vi "CONV 2D String Array to String.vi"(0 "2-D String":string[][](array[string]), 1 "Delimiters (,;)":string=",;") -> (6 "String":string)   [LabVIEW 2017]
doc: "This routine converts a 2-D String Array into a String list. There must be exactly 2 characters in the delimiters field. The first character is the Column Delimiter, and the second character is the Row Delimiter.\n\nExample:\n\n2-D String Input:\n\n1 2 3\n4 5 6\n\nDelimiters:\n,;\n\nString Output:\n\n1,2,3;4,5,6"
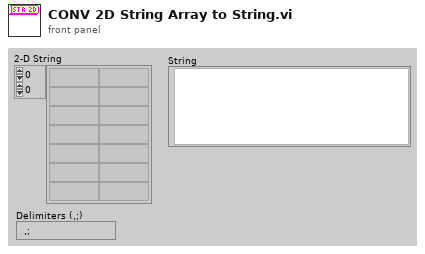
[diagram p1: front panel]
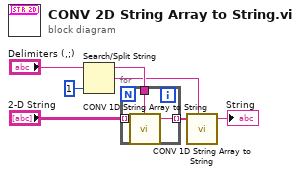
[diagram p0: block diagram]
diagram:
  n1 = Search/Split String(string="Delimiters (,;)", offset (0)=1) -> (substring before match=w2:string, match + rest of string=w1:string)  [unwired: 2 out]
  n2 = for {
    tunnel: "2-D String" -> [w10] mode=indexing
    tunnel: [w9] -> w6 mode=indexing
    tunnel: w2 -> [w8]
    n3 = call "CONV 1D String Array to String.vi"("1-D String"=w10, "Delimiter (,)"=w8) -> ("String"=w9:string)  [unwired: 7 out]
  }
  n4 = call "CONV 1D String Array to String.vi"("1-D String"=w6, "Delimiter (,)"=w1) -> ("String"=→"String":string)  [unwired: 7 out]
